vi "cont_string (SubVI).vi"(11 "cont":dbl[](array[numeric])) -> (3 "String":string)   [LabVIEW 2013]
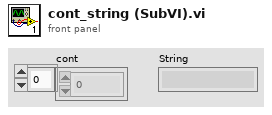
[diagram p1: front panel]
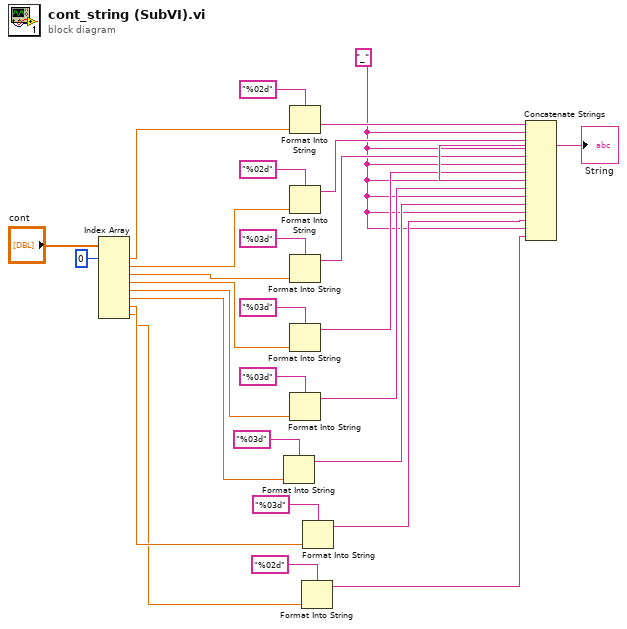
[diagram p0: block diagram]
diagram:
  w2 = "_" ("string")
  n1 = Index Array(array="cont", index #1=0 ("index")) -> (element #1=w14:dbl, element #2=w15:dbl, element #3=w16:dbl, element #4=w17:dbl, element #5=w18:dbl, element #6=w9:dbl, element #7=w5:dbl, element #8=w4:dbl)  [unwired: 7 in]
  n2 = Format Into String(format string="%03d", w9) -> (resulting string=w8:string)  [unwired: 2 in, 1 out]
  n3 = Format Into String(format string="%02d", w14) -> (resulting string=w19:string)  [unwired: 2 in, 1 out]
  n4 = Format Into String(format string="%02d", w15) -> (resulting string=w23:string)  [unwired: 2 in, 1 out]
  n5 = Format Into String(format string="%03d", w16) -> (resulting string=w22:string)  [unwired: 2 in, 1 out]
  n6 = Format Into String(format string="%03d", w17) -> (resulting string=w21:string)  [unwired: 2 in, 1 out]
  n7 = Format Into String(format string="%03d", w18) -> (resulting string=w20:string)  [unwired: 2 in, 1 out]
  n8 = Format Into String(format string="%02d", w4) -> (resulting string=w1:string)  [unwired: 2 in, 1 out]
  n9 = Format Into String(format string="%03d", w5) -> (resulting string=w3:string)  [unwired: 2 in, 1 out]
  n10 = Concatenate Strings(w19, w2, w23, w2, w22, w2, w21, w2, w20, w2, w8, w2, w3, w2, w1) -> (→"String":string)
